vi "BBoxOne.vi"() -> ()   [LabVIEW 2021]
uses:
  D:/tmytek/Source/bbox-api/windows example/BBoxOne Series/LabVIEW/BBoxAPI.dll
  BBoxAPI.dll
  kernel32.dll
panel:
  out "checkCaliTableLocation":bool
  out "Exists Table Filenames":string[](array[string])
  out "Get Current Working Directory":path
  in  "Set Current Working Directory":path
  in  "Target AAkit Index":u32
  in  "Target Freq Index":u32
  out "RX Board4 elementDR":dbl
  out "TX Board4  elementDR":dbl
  out "RX Board3 elementDR":dbl
  out "TX Board3 elementDR":dbl
  out "RX Board2 elementDR":dbl
  out "TX Board2 elementDR":dbl
  out "RX Board1 elementDR":dbl
  out "TX Board1 elementDR":dbl
  out "setAllChannelGain":i32
  in  "Board Number:\nRange from 1 to 4":i32=1
  in  "Board_Ch4_db":dbl step=0.5
  in  "Board_Ch3_db":dbl step=0.5
  in  "Board_Ch2_db":dbl step=0.5
  in  "Board_Ch1_db":dbl step=0.5
  out "readChannelSwitchValues":i32[][](array[numeric])
  out "Target Frequency":string
  out "Target AAKit Name":string
  out "getAAKitList":string[](array[string])
  out "RX MAX GAIN":dbl
  out "TX MAX GAIN":dbl
  out "setBeamAngle":i32(ring)=13 items=["OK"=0, "WARNING"=1, "ERROR"=2, "NO_RESPONSE"=3, "ERROR_GET_SN"=10, "ERROR_DEV_TYPE"=11, "ERROR_INIT_OBJECT"=12, "ERROR_DEV_NOT_INIT"=13, "ERROR_METHOD_NOT_FOUND"=14, "ERROR_REFLECTION"=15, "ERROR_POWER"=16, "ERROR_NETWORK_NOT_INIT"=20, "ERROR_NETWORK_INIT"=21, "ERROR_NETWORK_CONNECT_TIMEOUT"=22, "ERROR_DISCONNECT"=23, "ERROR_SOCKET"=24, "ERROR_SEND_CMD"=25, "ERROR_RESP_CMD"=26, "ERROR_DEV_COUNT_ZERO"=30, "ERROR_CMD"=40, "ERROR_CMD_INIT"=41, "ERROR_BF_AAKIT"=100, "ERROR_BF_NO_AAKIT"=101, "ERROR_BF_CALI_PATH"=102, "ERROR_BF_BEAMXY"=103, "ERROR_BF_GEN"=104, "ERROR_BF_TRMODE"=105, "STATUS_BF_LOAD_CALI_INCOMPLTE"=106, "ERROR_BF_LOAD_CALI_PARSE_FAILED"=107, "ERROR_FREQ_EQUATION"=250, "ERROR_PLO_CRC"=251, "WARNING_HARMONIC"=252, "ERROR_HARMONIC_BLOCK"=253]
  in  "Phi:\nRange from 0 to 359":i32=30 min=-45 max=45 step=1
  out "switchChannelPower":string
  in  "Power :\nON = 0 OFF = 1":i32
  out "selectAAKit":i32(ring) items=["OK"=0, "WARNING"=1, "ERROR"=2, "NO_RESPONSE"=3, "ERROR_GET_SN"=10, "ERROR_DEV_TYPE"=11, "ERROR_INIT_OBJECT"=12, "ERROR_DEV_NOT_INIT"=13, "ERROR_METHOD_NOT_FOUND"=14, "ERROR_REFLECTION"=15, "ERROR_POWER"=16, "ERROR_NETWORK_NOT_INIT"=20, "ERROR_NETWORK_INIT"=21, "ERROR_NETWORK_CONNECT_TIMEOUT"=22, "ERROR_DISCONNECT"=23, "ERROR_SOCKET"=24, "ERROR_SEND_CMD"=25, "ERROR_RESP_CMD"=26, "ERROR_DEV_COUNT_ZERO"=30, "ERROR_CMD"=40, "ERROR_CMD_INIT"=41, "ERROR_BF_AAKIT"=100, "ERROR_BF_NO_AAKIT"=101, "ERROR_BF_CALI_PATH"=102, "ERROR_BF_BEAMXY"=103, "ERROR_BF_GEN"=104, "ERROR_BF_TRMODE"=105, "STATUS_BF_LOAD_CALI_INCOMPLTE"=106, "ERROR_BF_LOAD_CALI_PARSE_FAILED"=107, "ERROR_FREQ_EQUATION"=250, "ERROR_PLO_CRC"=251, "WARNING_HARMONIC"=252, "ERROR_HARMONIC_BLOCK"=253]
  out "readBeamPhaseValues":i32[][](array[numeric])
  out "readBeamGainValues":dbl[][](array[numeric])
  in  "Theta:\nRange from 0 to 45":i32=15 min=-45 max=45 step=1
  in  "Beam Gain:\nIn tx_mode : \ntx_min_gain to tx_max_gain\nIn rx mode : \nrx_min_gain to to rx_max_gain":dbl=1.0 step=0.5
  out "setChannelGainPhase":string
  in  "deg range from 0 to 359":i32 min=0 max=355 step=5
  in  "db range:\nIn tx_mode : \ntx_min_gain to tx_max_gain\nIn rx mode : \nrx_min_gain to to rx_max_gain":dbl step=0.5
  in  "Channel:\n Range from 1 to 16":i32=16 min=1 max=16
  in  "Mode : \nTX = 1 \nRX = 2":i32=1 min=1 max=2 step=1
  out "RX MIN GAIN":dbl
  out "TX MIN GAIN":dbl
  out "Current Mode":i32
  out "SwitchTxRxMode":i32(ring) items=["OK"=0, "WARNING"=1, "ERROR"=2, "NO_RESPONSE"=3, "ERROR_GET_SN"=10, "ERROR_DEV_TYPE"=11, "ERROR_INIT_OBJECT"=12, "ERROR_DEV_NOT_INIT"=13, "ERROR_METHOD_NOT_FOUND"=14, "ERROR_REFLECTION"=15, "ERROR_POWER"=16, "ERROR_NETWORK_NOT_INIT"=20, "ERROR_NETWORK_INIT"=21, "ERROR_NETWORK_CONNECT_TIMEOUT"=22, "ERROR_DISCONNECT"=23, "ERROR_SOCKET"=24, "ERROR_SEND_CMD"=25, "ERROR_RESP_CMD"=26, "ERROR_DEV_COUNT_ZERO"=30, "ERROR_CMD"=40, "ERROR_CMD_INIT"=41, "ERROR_BF_AAKIT"=100, "ERROR_BF_NO_AAKIT"=101, "ERROR_BF_CALI_PATH"=102, "ERROR_BF_BEAMXY"=103, "ERROR_BF_GEN"=104, "ERROR_BF_TRMODE"=105, "STATUS_BF_LOAD_CALI_INCOMPLTE"=106, "ERROR_BF_LOAD_CALI_PARSE_FAILED"=107, "ERROR_FREQ_EQUATION"=250, "ERROR_PLO_CRC"=251, "WARNING_HARMONIC"=252, "ERROR_HARMONIC_BLOCK"=253]
  out "setOperatingFreq":i32(ring)=13 items=["OK"=0, "WARNING"=1, "ERROR"=2, "NO_RESPONSE"=3, "ERROR_GET_SN"=10, "ERROR_DEV_TYPE"=11, "ERROR_INIT_OBJECT"=12, "ERROR_DEV_NOT_INIT"=13, "ERROR_METHOD_NOT_FOUND"=14, "ERROR_REFLECTION"=15, "ERROR_POWER"=16, "ERROR_NETWORK_NOT_INIT"=20, "ERROR_NETWORK_INIT"=21, "ERROR_NETWORK_CONNECT_TIMEOUT"=22, "ERROR_DISCONNECT"=23, "ERROR_SOCKET"=24, "ERROR_SEND_CMD"=25, "ERROR_RESP_CMD"=26, "ERROR_DEV_COUNT_ZERO"=30, "ERROR_CMD"=40, "ERROR_CMD_INIT"=41, "ERROR_BF_AAKIT"=100, "ERROR_BF_NO_AAKIT"=101, "ERROR_BF_CALI_PATH"=102, "ERROR_BF_BEAMXY"=103, "ERROR_BF_GEN"=104, "ERROR_BF_TRMODE"=105, "STATUS_BF_LOAD_CALI_INCOMPLTE"=106, "ERROR_BF_LOAD_CALI_PARSE_FAILED"=107, "ERROR_FREQ_EQUATION"=250, "ERROR_PLO_CRC"=251, "WARNING_HARMONIC"=252, "ERROR_HARMONIC_BLOCK"=253]
  out "getFrequencyList":string[](array[string])
  out "Init":i32(ring)=13 items=["OK"=0, "WARNING"=1, "ERROR"=2, "NO_RESPONSE"=3, "ERROR_GET_SN"=10, "ERROR_DEV_TYPE"=11, "ERROR_INIT_OBJECT"=12, "ERROR_DEV_NOT_INIT"=13, "ERROR_METHOD_NOT_FOUND"=14, "ERROR_REFLECTION"=15, "ERROR_POWER"=16, "ERROR_NETWORK_NOT_INIT"=20, "ERROR_NETWORK_INIT"=21, "ERROR_NETWORK_CONNECT_TIMEOUT"=22, "ERROR_DISCONNECT"=23, "ERROR_SOCKET"=24, "ERROR_SEND_CMD"=25, "ERROR_RESP_CMD"=26, "ERROR_DEV_COUNT_ZERO"=30, "ERROR_CMD"=40, "ERROR_CMD_INIT"=41, "ERROR_BF_AAKIT"=100, "ERROR_BF_NO_AAKIT"=101, "ERROR_BF_CALI_PATH"=102, "ERROR_BF_BEAMXY"=103, "ERROR_BF_GEN"=104, "ERROR_BF_TRMODE"=105, "STATUS_BF_LOAD_CALI_INCOMPLTE"=106, "ERROR_BF_LOAD_CALI_PARSE_FAILED"=107, "ERROR_FREQ_EQUATION"=250, "ERROR_PLO_CRC"=251, "WARNING_HARMONIC"=252, "ERROR_HARMONIC_BLOCK"=253]
  out "SN":string
  out "ScanningDevice":string[](array[string])
  # "Notice:\n\nThe Set / Get Current Working Diectory Path must be \nthe sample code directory path\n\nbbox-api\\example\\BBoxOne Series\\LabVIEW\\\n\nand must exist\n\nbbox-api\\example\\BBoxOne Series\\LabVIEW\\BBoxAPI.dll\n\nbbox-api\\example\\BBoxOne Series\\LabVIEW\\files\\\n\nbbox-api\\example\\BBoxOne Series\\LabVIEW\\logs\\\n\n---\n\n1. setChannelGainPhase(int board, int ch, double db, int deg,string sn)\n \n  The formula of channel number(1 ~ 16) to board (1 ~ 4) and ch (1 ~ 4) :\n\n   (1) board = ((channel number - 1) / 4) + 1\n   (2) ch = ((channel number - 1) % 4) +1\n\n---\n\n2. setAllChannelGain(int board, double ch1_db,double ch2_db,double ch3_db, double ch4_db, string sn)\n\n  The channel gain settings on the same board should not exceed the board elementDR. \n\n   (1) board = ((channel number - 1) / 4) + 1\n   (2) Example\n           - board = 1\n           - TX DR = (-5.5 db to 10.5 db) \n           - TX elementDR =   4.5 db\n\n            - Valid Settings :\n               ch1_db = 10.5 db\n               ch2_db = 6 db\n               ch3_db = 10 db\n               ch4_db = 8 db  \n\n\n            - Invalid Settings (ch1_db and ch2_db exceed 4.5 db):\n               ch1_db = 10.5 db\n               ch2_db = 5.5 db\n               ch3_db = 10 db\n               ch4_db = 8 db  \n\n---\n\n3. Channel order on GUI  in labview and TMXLab Kits s different.\n\n\n(1) TMXLAB Kits GUI Channel Order\n\nCh04  Ch03  Ch02  Ch01\n\nCh08  Ch07  Ch06  Ch05\n\nCh12  Ch11  Ch10  Ch09\n\nCh16  Ch15  Ch14  Ch13\n\n\n\n(2) Labview GUI Channel Order\n\nCh01  Ch02  Ch03  Ch04\n\nCh05  Ch06  Ch07  Ch08\n\nCh09  Ch10  Ch11  Ch12\n\nCh13  Ch14  Ch15  Ch16"
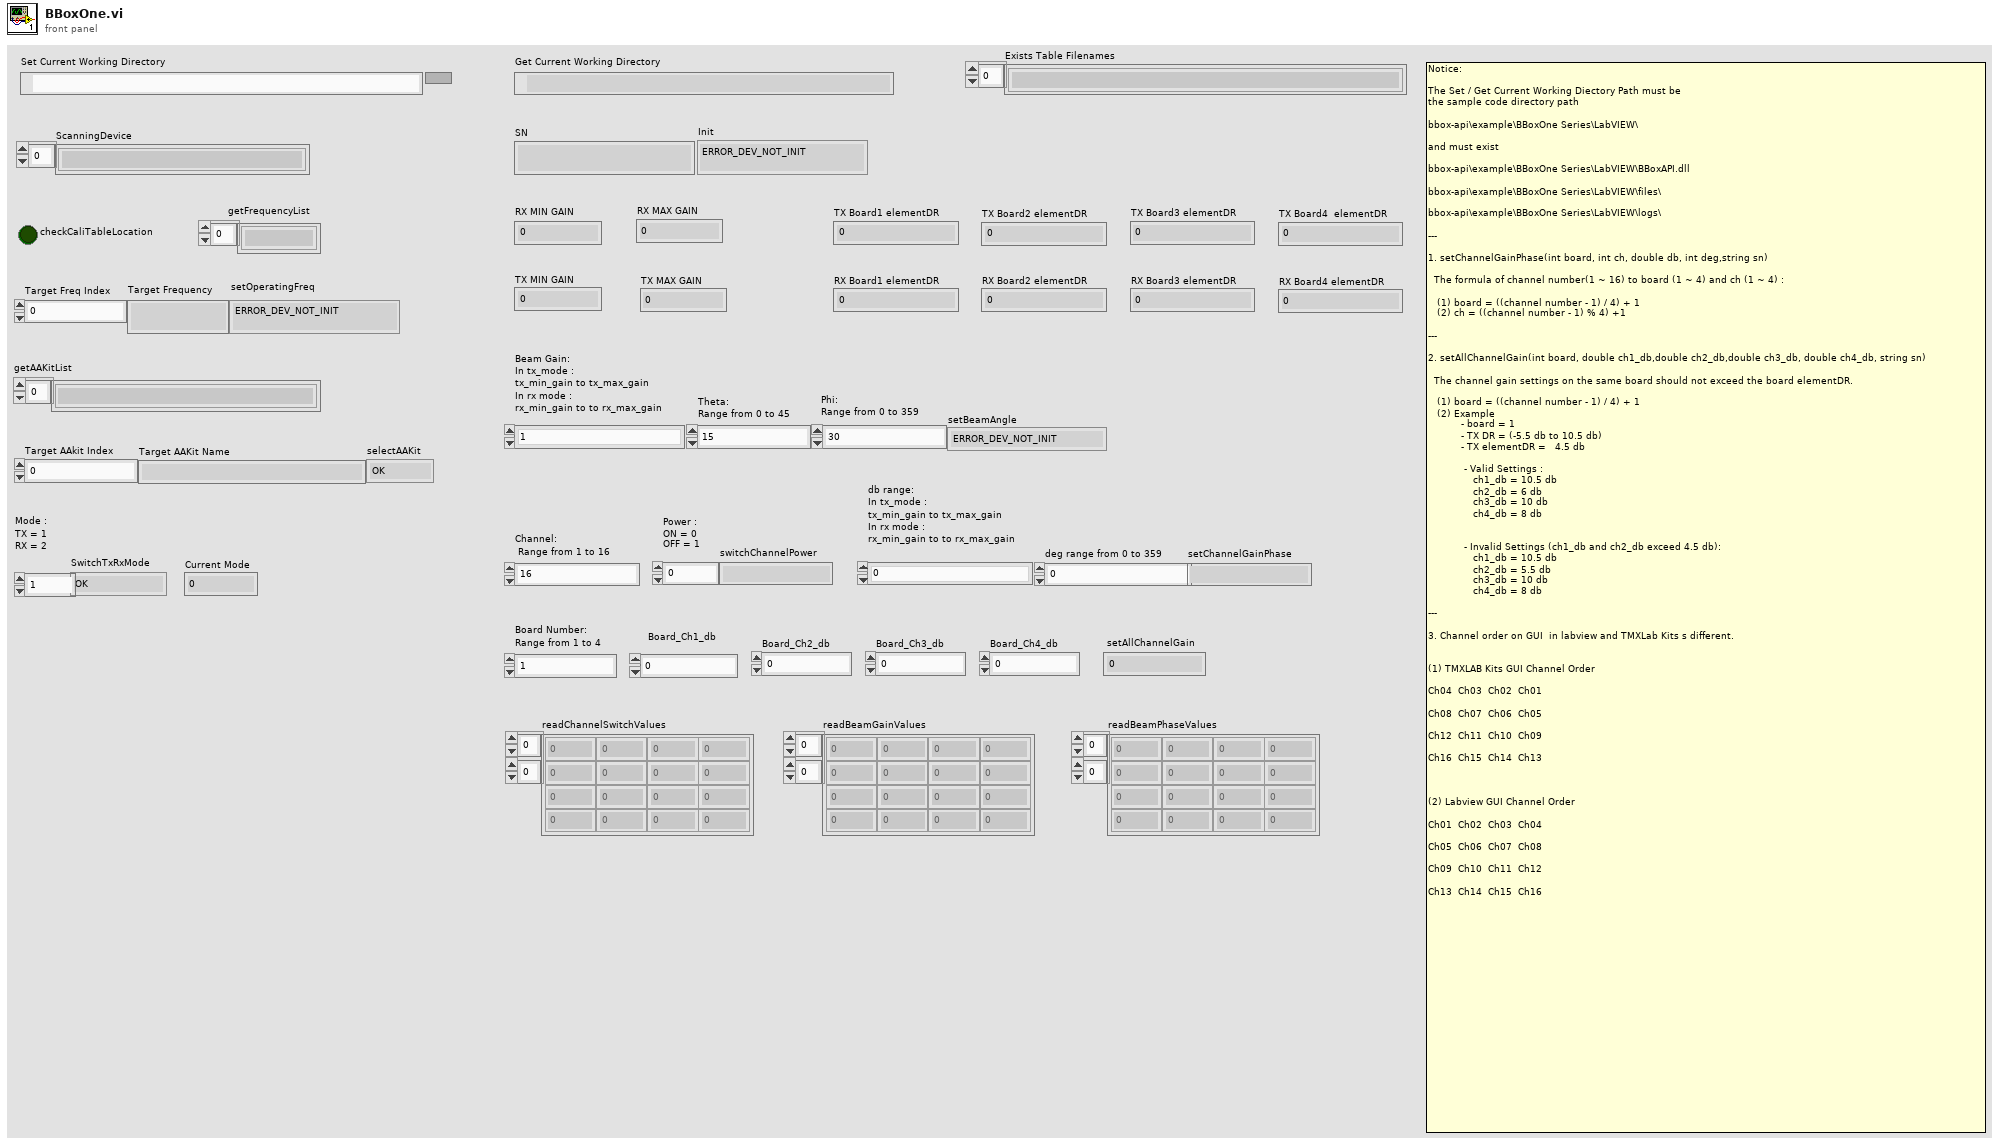
[diagram p1: front panel]
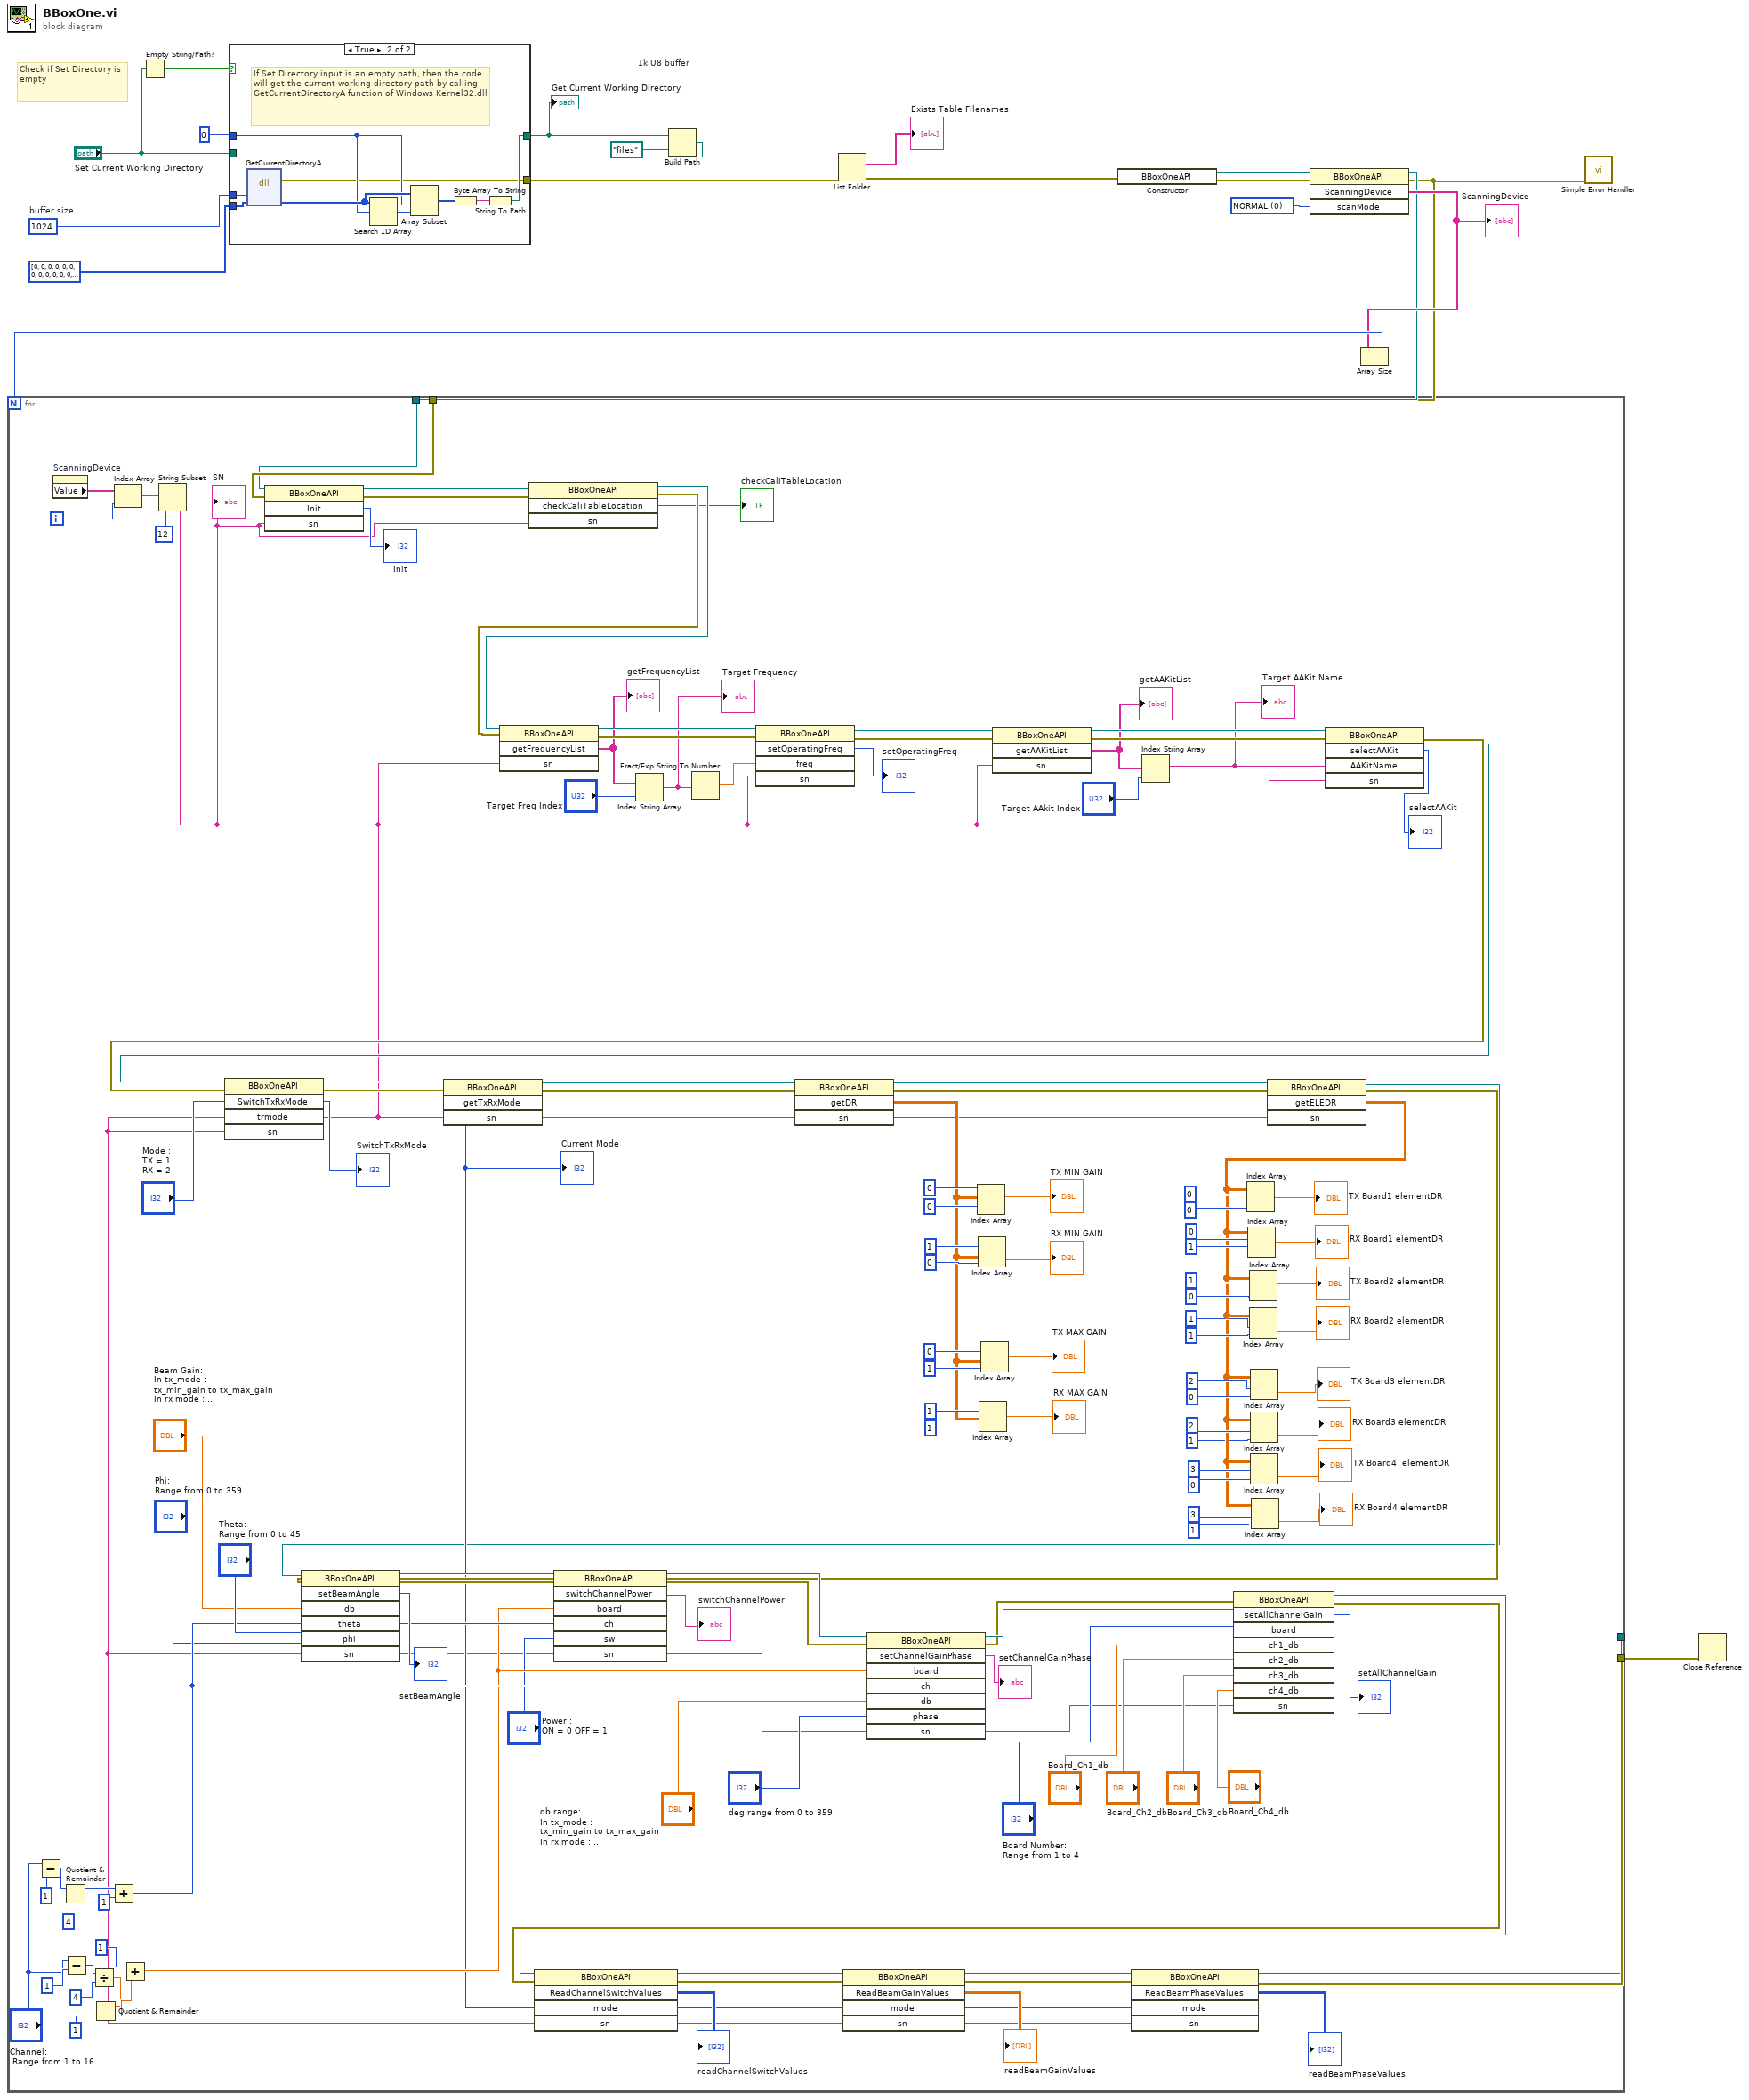
[diagram p0: block diagram]
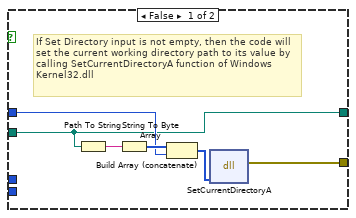
[diagram p2: hidden frame]
diagram:
  w9 = 1024  # buffer size
  w8 = u8[] [0, 0, 0, 0, 0, 0, 0, 0, 0, 0, 0, 0, 0, 0, 0, 0, 0, 0, 0, 0, 0, 0, 0, 0, 0, 0, 0, 0, 0, 0, 0, 0, 0, 0, 0, 0, 0, 0, 0, 0, 0, 0, 0, 0, 0, 0, 0, 0, 0, 0, 0, 0, 0, 0, 0, 0, 0, 0, 0, 0, 0, 0, 0, 0, 0, 0, 0, 0, 0, 0, 0, 0, 0, 0, 0, 0, 0, 0, 0, 0, 0, 0, 0, 0, 0, 0, 0, 0, 0, 0, 0, 0, 0, 0, 0, 0, 0, 0, 0, 0, 0, 0, 0, 0, 0, 0, 0, 0, 0, 0, 0, 0, 0, 0, 0, 0, 0, 0, 0, 0, 0, 0, 0, 0, 0, 0, 0, 0, 0, 0, 0, 0, 0, 0, 0, 0, 0, 0, 0, 0, 0, 0, 0, 0, 0, 0, 0, 0, 0, 0, 0, 0, 0, 0, 0, 0, 0, 0, 0, 0, 0, 0, 0, 0, 0, 0, 0, 0, 0, 0, 0, 0, 0, 0, 0, 0, 0, 0, 0, 0, 0, 0, 0, 0, 0, 0, 0, 0, 0, 0, 0, 0, 0, 0, 0, 0, 0, 0, 0, 0, 0, 0, 0, 0, 0, 0, 0, 0, 0, 0, 0, 0, 0, 0, 0, 0, 0, 0, 0, 0, 0, 0, 0, 0, 0, 0, 0, 0, 0, 0, 0, 0, 0, 0, 0, 0, 0, 0, 0, 0, 0, 0, 0, 0, 0, 0, 0, 0, 0, 0, 0, 0, 0, 0, 0, 0, 0, 0, 0, 0, 0, 0, 0, 0, 0, 0, 0, 0, 0, 0, 0, 0, 0, 0, 0, 0, 0, 0, 0, 0, 0, 0, 0, 0, 0, 0, 0, 0, 0, 0, 0, 0, 0, 0, 0, 0, 0, 0, 0, 0, 0, 0, 0, 0, 0, 0, 0, 0, 0, 0, 0, 0, 0, 0, 0, 0, 0, 0, 0, 0, 0, 0, 0, 0, 0, 0, 0, 0, 0, 0, 0, 0, 0, 0, 0, 0, 0, 0, 0, 0, 0, 0, 0, 0, 0, 0, 0, 0, 0, 0, 0, 0, 0, 0, 0, 0, 0, 0, 0, 0, 0, 0, 0, 0, 0, 0, 0, 0, 0, 0, 0, 0, 0, 0, 0, 0, 0, 0, 0, 0, 0, 0, 0, 0, 0, 0, 0, 0, 0, 0, 0, 0, 0, 0, 0, 0, 0, 0, 0, 0, 0, 0, 0, 0, 0, 0, 0, 0, 0, 0, 0, 0, 0, 0, 0, 0, 0, 0, 0, 0, 0, 0, 0, 0, 0, 0, 0, 0, 0, 0, 0, 0, 0, 0, 0, 0, 0, 0, 0, 0, 0, 0, 0, 0, 0, 0, 0, 0, 0, 0, 0, 0, 0, 0, 0, 0, 0, 0, 0, 0, 0, 0, 0, 0, 0, 0, 0, 0, 0, 0, 0, 0, 0, 0, 0, 0, 0, 0, 0, 0, 0, 0, 0, 0, 0, 0, 0, 0, 0, 0, 0, 0, 0, 0, 0, 0, 0, 0, 0, 0, 0, 0, 0, 0, 0, 0, 0, 0, 0, 0, 0, 0, 0, 0, 0, 0, 0, 0, 0, 0, 0, 0, 0, 0, 0, 0, 0, 0, 0, 0, 0, 0, 0, 0, 0, 0, 0, 0, 0, 0, 0, 0, 0, 0, 0, 0, 0, 0, 0, 0, 0, 0, 0, 0, 0, 0, 0, 0, 0, 0, 0, 0, 0, 0, 0, 0, 0, 0, 0, 0, 0, 0, 0, 0, 0, 0, 0, 0, 0, 0, 0, 0, 0, 0, 0, 0, 0, 0, 0, 0, 0, 0, 0, 0, 0, 0, 0, 0, 0, 0, 0, 0, 0, 0, 0, 0, 0, 0, 0, 0, 0, 0, 0, 0, 0, 0, 0, 0, 0, 0, 0, 0, 0, 0, 0, 0, 0, 0, 0, 0, 0, 0, 0, 0, 0, 0, 0, 0, 0, 0, 0, 0, 0, 0, 0, 0, 0, 0, 0, 0, 0, 0, 0, 0, 0, 0, 0, 0, 0, 0, 0, 0, 0, 0, 0, 0, 0, 0, 0, 0, 0, 0, 0, 0, 0, 0, 0, 0, 0, 0, 0, 0, 0, 0, 0, 0, 0, 0, 0, 0, 0, 0, 0, 0, 0, 0, 0, 0, 0, 0, 0, 0, 0, 0, 0, 0, 0, 0, 0, 0, 0, 0, 0, 0, 0, 0, 0, 0, 0, 0, 0, 0, 0, 0, 0, 0, 0, 0, 0, 0, 0, 0, 0, 0, 0, 0, 0, 0, 0, 0, 0, 0, 0, 0, 0, 0, 0, 0, 0, 0, 0, 0, 0, 0, 0, 0, 0, 0, 0, 0, 0, 0, 0, 0, 0, 0, 0, 0, 0, 0, 0, 0, 0, 0, 0, 0, 0, 0, 0, 0, 0, 0, 0, 0, 0, 0, 0, 0, 0, 0, 0, 0, 0, 0, 0, 0, 0, 0, 0, 0, 0, 0, 0, 0, 0, 0, 0, 0, 0, 0, 0, 0, 0, 0, 0, 0, 0, 0, 0, 0, 0, 0, 0, 0, 0, 0, 0, 0, 0, 0, 0, 0, 0, 0, 0, 0, 0, 0, 0, 0, 0, 0, 0, 0, 0, 0, 0, 0, 0, 0, 0, 0, 0, 0, 0, 0, 0, 0, 0, 0, 0, 0, 0, 0, 0, 0, 0, 0, 0, 0, 0, 0, 0, 0, 0, 0, 0, 0, 0, 0, 0, 0, 0, 0, 0, 0, 0, 0, 0, 0, 0, 0, 0, 0, 0, 0, 0, 0, 0, 0, 0, 0, 0, 0, 0, 0, 0, 0, 0, 0, 0, 0, 0, 0, 0, 0, 0, 0, 0, 0, 0, 0, 0, 0, 0, 0, 0, 0, 0, 0, 0, 0, 0, 0, 0, 0, 0, 0, 0, 0, 0, 0, 0, 0, 0, 0, 0, 0, 0, 0, 0, 0, 0, 0, 0, 0, 0, 0, 0, 0, 0, 0, 0, 0, 0, 0, 0, 0, 0, 0, 0, 0, 0, 0, 0, 0, 0, 0, 0, 0, 0, 0, 0, 0, 0, 0, 0, 0, 0, 0, 0, 0, 0, 0, 0, 0, 0, 0, 0, 0, 0, 0, 0, 0, 0, 0, 0, 0, 0, 0, 0, 0, 0, 0, 0, 0, 0, 0, 0, 0, 0, 0, 0, 0]  # 1k U8 buffer
  w20 = 0 items=["NORMAL", "FAST"] ("scanMode")
  # "Check if Set Directory is empty"
  n1 = Empty String/Path?(string/path="Set Current Working Directory") -> (empty?=w10:bool)
  n2 = case shown="True" w10 {
    tunnel: "Set Current Working Directory" -> [w22 _]
    tunnel: u8 0 -> [w24 w31]
    tunnel: w9 -> [_ w30]
    tunnel: w8 -> [_ w29]
    tunnel: [w22 w28] -> w3
    tunnel: [w21 w27] -> w6
    frame False {
      # "If Set Directory input is not empty, then the code will set the current working directory path to its value by calling SetCurrentDirectoryA function of Windows Kernel32.dll"
      n3 = Path To String(path=w22) -> (string=w23:string)
      n4 = String To Byte Array(string=w23) -> (unsigned byte array=w26:u8[])
      n5 = Build Array (concatenate)(w26, w24) -> (w25:u8[])
      n6 = dll-call lib="Kernel32.dll" fn="SetCurrentDirectoryA" label="Kernel32.dll - \nSetCurrentDirectoryA"("lpPathName"=w25) -> (error out=w21:errorcluster)  [unwired: 4 in, 2 out]
    }
    frame True {
      # "If Set Directory input is an empty path, then the code will get the current working directory path by calling GetCurrentDirectoryA function of Windows Kernel32.dll"
      n7 = dll-call lib="kernel32.dll" fn="GetCurrentDirectoryA" label="Kernel32.dll - \nGetCurrentDirectoryA"("nBufferLength"=w30, "lpBuffer"=w29) -> (error out=w27:errorcluster, "lpBuffer"=w34:u8[])  [unwired: 4 in, 2 out]
      n8 = Search 1D Array(1D array=w34, element=w31) -> (index of element=w35:i32)  [unwired: 1 out]
      n9 = Array Subset(array=w34, index=w31, length=w35) -> (w32:u8[])
      n10 = Byte Array To String(unsigned byte array=w32) -> (string=w33:string)
      n11 = String To Path(string=w33) -> (path=w28:path)
    }
  }
  "Get Current Working Directory" <- w3
  n12 = Build Path(base path=w3, name or relative path=path "files") -> (appended path=w1:path)
  n13 = List Folder(path=w1, error in=w6) -> (filenames=→"Exists Table Filenames":string[], error out=w5:errorcluster)  [unwired: 2 in, 2 out]
  n14 = constructor class="BBoxOneAPI"(error in=w5) -> (reference out=w19:refnum<k24>, error out=w18:errorcluster)  [unwired: 2 in, 1 out]
  n15 = invoke class="BBoxOneAPI" method="ScanningDevice"(reference=w19, error in=w18, "scanMode"=w20) -> (reference out=w15:refnum<k24>, error out=w14:errorcluster, "ScanningDevice"=w16:string[])  [unwired: 1 in, 1 out]
  "ScanningDevice" <- w16
  n16 = Array Size(array=w16) -> (size(s)=w17:i32)
  n17 = for {
    N: w17 -> [_]
    tunnel: w15 -> [w130]
    tunnel: w14 -> [w159]
    tunnel: [w45] -> w13
    tunnel: [w44] -> w12
    i -> [w72]
    n18 = Subtract(x="Channel:\n Range from 1 to 16", y=1) -> (x-y=w105:i32)
    n19 = property on="ScanningDevice" class="Arr (strict)"() -> ("Value"=w137:string[])  [unwired: 2 in, 2 out]
    n20 = Quotient & Remainder(x=w105, y=4) -> (x-y*floor(x/y)=w103:i32)  [unwired: 1 out]
    n21 = Subtract(x="Channel:\n Range from 1 to 16", y=1) -> (x-y=w116:i32)
    n22 = Divide(x=w116, y=4) -> (x/y=w109:dbl)
    n23 = Quotient & Remainder(x=w109, y=1) -> (floor(x/y)=w112:dbl)  [unwired: 1 out]
    n24 = Add(x=w103, y=1) -> (x+y=w111:i32)
    n25 = Index Array(array=w137, index=w72) -> (element=w161:string)
    n26 = Add(x=1, y=w112) -> (x+y=w110:dbl)
    n27 = String Subset(string=w161, length (rest)=12) -> (substring=w36:string)  [unwired: 1 in]
    "SN" <- w36
    n28 = invoke class="BBoxOneAPI" method="Init"(reference=w130, error in=w159, "sn"=w36) -> (reference out=w41:refnum<k24>, error out=w40:errorcluster, "Init"=→"Init":i32)  [unwired: 1 in, 1 out]
    n29 = invoke class="BBoxOneAPI" method="checkCaliTableLocation"(reference=w41, error in=w40, "sn"=w36) -> (reference out=w39:refnum<k24>, error out=w38:errorcluster, "checkCaliTableLocation"=→"checkCaliTableLocation":bool)  [unwired: 1 in, 1 out]
    n30 = invoke class="BBoxOneAPI" method="getFrequencyList"(reference=w39, error in=w38, "sn"=w36) -> (reference out=w136:refnum<k24>, error out=w135:errorcluster, "getFrequencyList"=w127:string[])  [unwired: 1 in, 1 out]
    "getFrequencyList" <- w127
    n31 = Index String Array(1:"Target Freq Index", 2:w127) -> (0:w123:string)  [unwired: 1 in]
    "Target Frequency" <- w123
    n32 = Fract/Exp String To Number(string=w123) -> (number=w128:dbl)  [unwired: 3 in, 1 out]
    n33 = invoke class="BBoxOneAPI" method="setOperatingFreq"(reference=w136, error in=w135, "freq"=w128, "sn"=w36) -> (reference out=w141:refnum<k24>, error out=w140:errorcluster, "setOperatingFreq"=→"setOperatingFreq":i32)  [unwired: 1 in, 2 out]
    n34 = invoke class="BBoxOneAPI" method="getAAKitList"(reference=w141, error in=w140, "sn"=w36) -> (reference out=w139:refnum<k24>, error out=w138:errorcluster, "getAAKitList"=w125:string[])  [unwired: 1 in, 1 out]
    "getAAKitList" <- w125
    n35 = Index String Array(1:"Target AAkit Index", 2:w125) -> (0:w124:string)  [unwired: 1 in]
    "Target AAKit Name" <- w124
    n36 = invoke class="BBoxOneAPI" method="selectAAKit"(reference=w139, error in=w138, "AAKitName"=w124, "sn"=w36) -> (reference out=w129:refnum<k24>, error out=w132:errorcluster, "selectAAKit"=→"selectAAKit":i32)  [unwired: 1 in, 2 out]
    n37 = invoke class="BBoxOneAPI" method="SwitchTxRxMode"(reference=w129, error in=w132, "trmode"="Mode : \nTX = 1 \nRX = 2", "sn"=w36) -> (reference out=w156:refnum<k24>, error out=w155:errorcluster, "SwitchTxRxMode"=→"SwitchTxRxMode":i32)  [unwired: 1 in, 2 out]
    n38 = invoke class="BBoxOneAPI" method="getTxRxMode"(reference=w156, error in=w155, "sn"=w36) -> (reference out=w154:refnum<k24>, error out=w153:errorcluster, "getTxRxMode"=w46:i32)  [unwired: 1 in, 1 out]
    "Current Mode" <- w46
    n39 = invoke class="BBoxOneAPI" method="getDR"(reference=w154, error in=w153, "sn"=w36) -> (reference out=w77:refnum<k24>, error out=w76:errorcluster, "getDR"=w43:dbl[][])  [unwired: 1 in, 1 out]
    n40 = Index Array(array=w43, index (row)=0, index (col)=0) -> (element=→"TX MIN GAIN":dbl)
    n41 = Index Array(array=w43, index (row)=1, index (col)=0) -> (element=→"RX MIN GAIN":dbl)
    n42 = Index Array(array=w43, index (row)=1, index (col)=1) -> (element=→"RX MAX GAIN":dbl)
    n43 = Index Array(array=w43, index (row)=0, index (col)=1) -> (element=→"TX MAX GAIN":dbl)
    n44 = invoke class="BBoxOneAPI" method="getELEDR"(reference=w77, error in=w76, "sn"=w36) -> (reference out=w42:refnum<k24>, error out=w75:errorcluster, "getELEDR"=w49:dbl[][])  [unwired: 1 in, 1 out]
    n45 = invoke class="BBoxOneAPI" method="setBeamAngle"(reference=w42, error in=w75, "db"="Beam Gain:\nIn tx_mode : \ntx_min_gain to tx_max_gain\nIn rx mode : \nrx_min_gain to to rx_max_gain", "theta"="Theta:\nRange from 0 to 45", "phi"="Phi:\nRange from 0 to 359", "sn"=w36) -> (reference out=w96:refnum<k24>, error out=w95:errorcluster, "setBeamAngle"=→"setBeamAngle":i32)  [unwired: 1 in, 4 out]
    n46 = invoke class="BBoxOneAPI" method="switchChannelPower"(reference=w96, error in=w95, "board"=w110, "ch"=w111, "sw"="Power :\nON = 0 OFF = 1", "sn"=w36) -> (reference out=w94:refnum<k24>, error out=w93:errorcluster, "switchChannelPower"=→"switchChannelPower":string)  [unwired: 1 in, 4 out]
    n47 = invoke class="BBoxOneAPI" method="setChannelGainPhase"(reference=w94, error in=w93, "board"=w110, "ch"=w111, "db"="db range:\nIn tx_mode : \ntx_min_gain to tx_max_gain\nIn rx mode : \nrx_min_gain to to rx_max_gain", "phase"="deg range from 0 to 359", "sn"=w36) -> (reference out=w86:refnum<k24>, error out=w85:errorcluster, "setChannelGainPhase"=→"setChannelGainPhase":string)  [unwired: 1 in, 5 out]
    n48 = invoke class="BBoxOneAPI" method="setAllChannelGain"(reference=w86, error in=w85, "board"="Board Number:\nRange from 1 to 4", "ch1_db"="Board_Ch1_db", "ch2_db"="Board_Ch2_db", "ch3_db"="Board_Ch3_db", "ch4_db"="Board_Ch4_db", "sn"=w36) -> (reference out=w84:refnum<k24>, error out=w83:errorcluster, "setAllChannelGain"=→"setAllChannelGain":i32)  [unwired: 1 in, 6 out]
    n49 = invoke class="BBoxOneAPI" method="ReadChannelSwitchValues"(reference=w84, error in=w83, "mode"=w46, "sn"=w36) -> (reference out=w82:refnum<k24>, error out=w81:errorcluster, "ReadChannelSwitchValues"=→"readChannelSwitchValues":i32[][])  [unwired: 1 in, 2 out]
    n50 = invoke class="BBoxOneAPI" method="ReadBeamGainValues"(reference=w82, error in=w81, "mode"=w46, "sn"=w36) -> (reference out=w80:refnum<k24>, error out=w79:errorcluster, "ReadBeamGainValues"=→"readBeamGainValues":dbl[][])  [unwired: 1 in, 2 out]
    n51 = invoke class="BBoxOneAPI" method="ReadBeamPhaseValues"(reference=w80, error in=w79, "mode"=w46, "sn"=w36) -> (reference out=w44:refnum<k24>, error out=w45:errorcluster, "ReadBeamPhaseValues"=→"readBeamPhaseValues":i32[][])  [unwired: 1 in, 2 out]
    n52 = Index Array(array=w49, index (row)=0, index (col)=0) -> (element=→"TX Board1 elementDR":dbl)
    n53 = Index Array(array=w49, index (row)=0, index (col)=1) -> (element=→"RX Board1 elementDR":dbl)
    n54 = Index Array(array=w49, index (row)=1, index (col)=0) -> (element=→"TX Board2 elementDR":dbl)
    n55 = Index Array(array=w49, index (row)=1, index (col)=1) -> (element=→"RX Board2 elementDR":dbl)
    n56 = Index Array(array=w49, index (row)=2, index (col)=0) -> (element=→"TX Board3 elementDR":dbl)
    n57 = Index Array(array=w49, index (row)=2, index (col)=1) -> (element=→"RX Board3 elementDR":dbl)
    n58 = Index Array(array=w49, index (row)=3, index (col)=0) -> (element=→"TX Board4  elementDR":dbl)
    n59 = Index Array(array=w49, index (row)=3, index (col)=1) -> (element=→"RX Board4 elementDR":dbl)
  }
  n60 = call <vilib>:"Simple Error Handler.vi"("error in (no error)"=w14) -> ()  [unwired: 4 in, 5 out]
  n61 = Close Reference(reference=w12, error in (no error)=w13) -> ()  [unwired: 1 out]
